vi "3-lorentzian-heat-response -- analytic derivatives.vi"(0 "ζ":dbl(slide)=0.000285 min=0.0 max=0.3 step=1e-06 scale=0.01..10.0 scale format="%#_3p", 1 "T1":dbl(slide)=0.000285 min=0.0 max=0.3 step=1e-06 scale=0.01..10.0 scale format="%#_3p", 2 "τS":dbl(slide)=0.000285 min=0.0 max=0.3 step=1e-06 scale=0.01..10.0 scale format="%#_3p", 3 "τN":dbl(slide)=0.000285 min=0.0 max=0.3 step=1e-06 scale=0.01..10.0 scale format="%#_3p", 4 "τC":dbl(slide)=0.000285 min=0.0 max=0.3 step=1e-06 scale=0.01..10.0 scale format="%#_3p", 5 "κ0":dbl(slide)=0.000285 min=0.0 max=0.3 step=1e-06 scale=0.01..10.0 scale format="%#_3p", 7 "ω (rad/sec)":dbl=0.1 format="%#_10f", 8 "action":T1) -> (13 "R(ω)":cdb=0.1+0.0i format="%#_10f", 14 "d R(ω) / dζ":cdb=-1.0+0.0i, 15 "d R(ω) /  dT1":cdb=-1.0+0.0i, 16 "d R(ω) /  d τS":cdb=-1.0+0.0i, 17 "d R(ω) /  d τN":cdb=-1.0+0.0i, 18 "d R(ω) /  d τC":cdb=-1.0+0.0i, 19 "d R(ω) /  d κ0":cdb=-1.0+0.0i)   [LabVIEW 2020]
uses:
  3-lorentzian-heat-response action.ctl
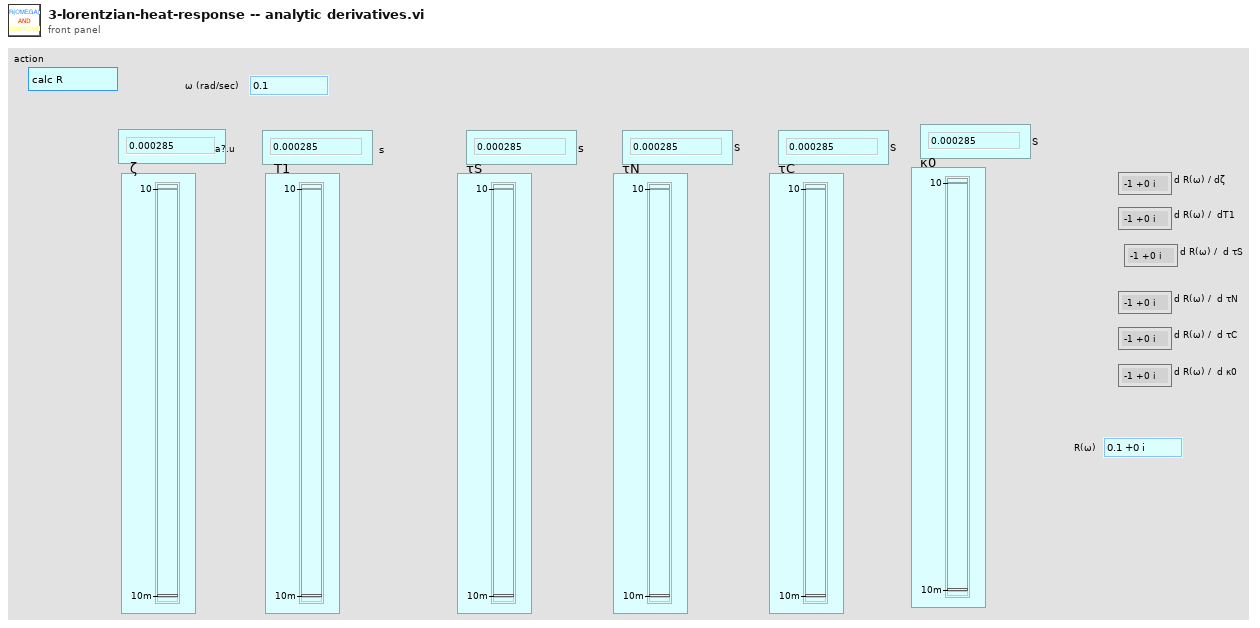
[diagram p1: front panel]
types:
  T1 = typedef "3-lorentzian-heat-response action.ctl" = enum16{"calc R", "create string", "calc m1m2m3", "dζ", "dT1", "dτS", "dτN", "dτC", "d-all", "dκ0"}
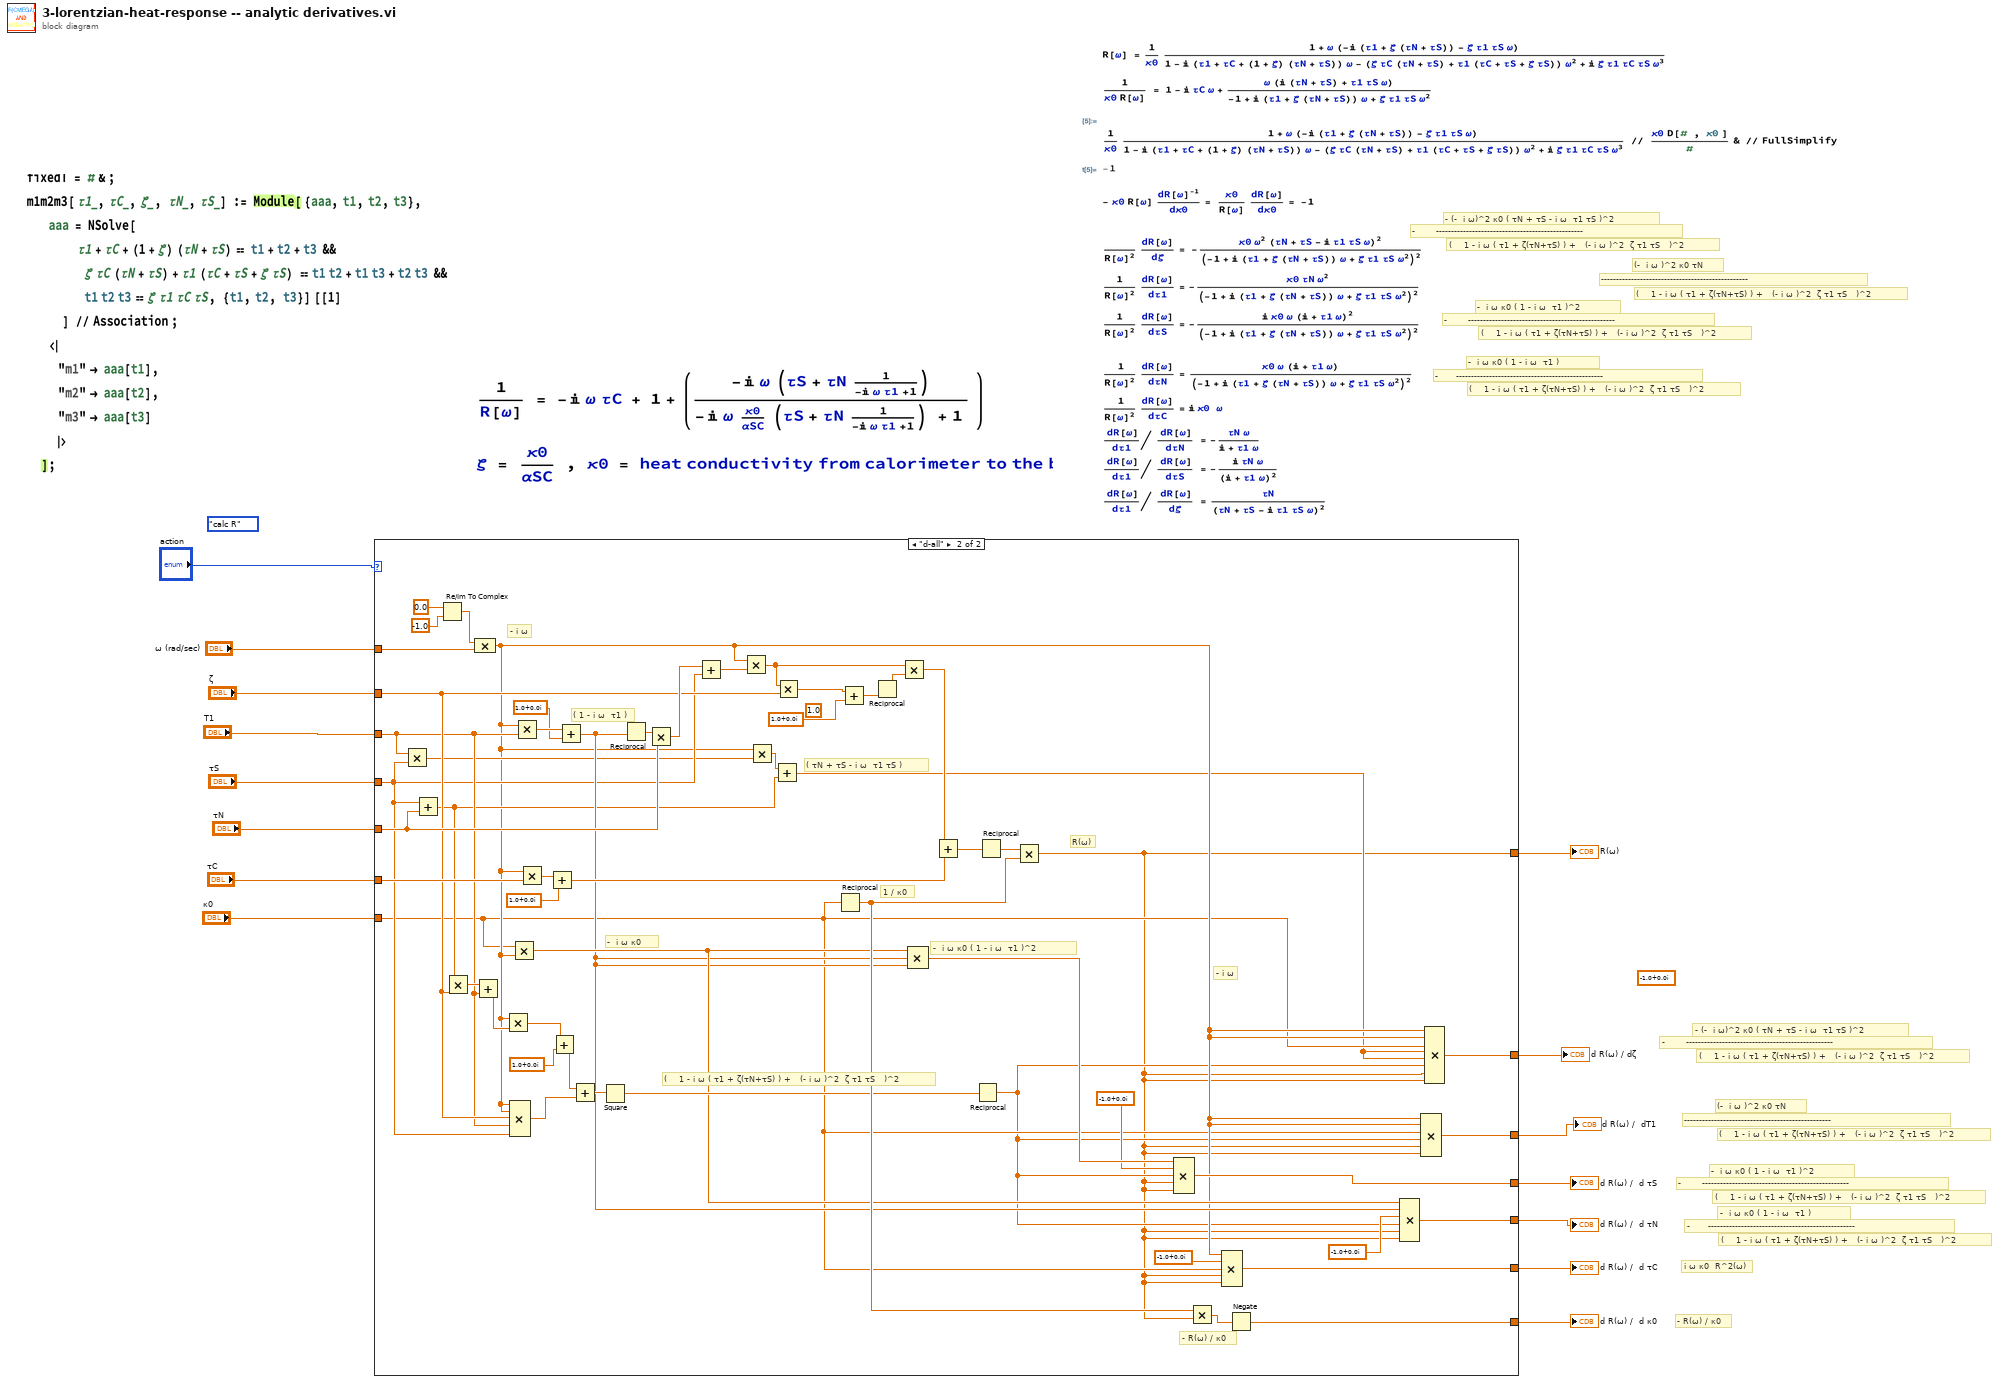
[diagram p0: block diagram]
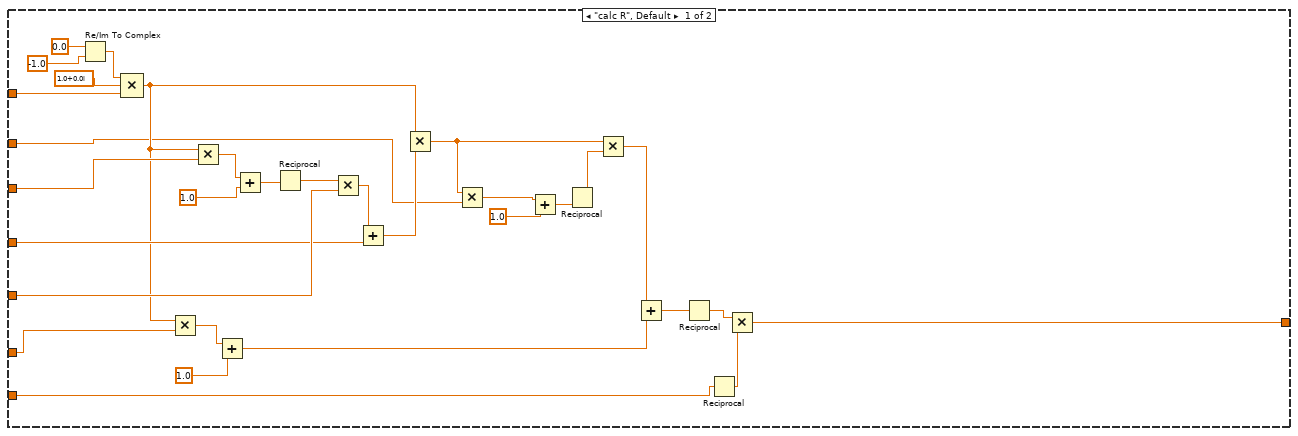
[diagram p2: hidden frame]
diagram:
  (unwired) cdb -1.0+0.0i ("value")
  (unwired) 3-lorentzian-heat-response_action."calc R" ("action")
  # "-       -------------------------------------------------"
  # "- (-  i ω)^2 κ0 ( τN + τS - i ω  τ1 τS )^2"
  # "(    1 - i ω ( τ1 + ζ(τN+τS) ) +   (- i ω )^2  ζ τ1 τS   )^2"
  # "-       -------------------------------------------------"
  # "-  i ω κ0 ( 1 - i ω  τ1 )^2"
  # "(    1 - i ω ( τ1 + ζ(τN+τS) ) +   (- i ω )^2  ζ τ1 τS   )^2"
  # "-------------------------------------------------"
  # "(-  i ω )^2 κ0 τN"
  # "(    1 - i ω ( τ1 + ζ(τN+τS) ) +   (- i ω )^2  ζ τ1 τS   )^2"
  # "-      -------------------------------------------------"
  # "-  i ω κ0 ( 1 - i ω  τ1 )"
  # "(    1 - i ω ( τ1 + ζ(τN+τS) ) +   (- i ω )^2  ζ τ1 τS   )^2"
  # "-       -------------------------------------------------"
  # "- (-  i ω)^2 κ0 ( τN + τS - i ω  τ1 τS )^2"
  # "(    1 - i ω ( τ1 + ζ(τN+τS) ) +   (- i ω )^2  ζ τ1 τS   )^2"
  # "-------------------------------------------------"
  # "(-  i ω )^2 κ0 τN"
  # "(    1 - i ω ( τ1 + ζ(τN+τS) ) +   (- i ω )^2  ζ τ1 τS   )^2"
  # "-      -------------------------------------------------"
  # "-  i ω κ0 ( 1 - i ω  τ1 )"
  # "(    1 - i ω ( τ1 + ζ(τN+τS) ) +   (- i ω )^2  ζ τ1 τS   )^2"
  # "-       -------------------------------------------------"
  # "-  i ω κ0 ( 1 - i ω  τ1 )^2"
  # "(    1 - i ω ( τ1 + ζ(τN+τS) ) +   (- i ω )^2  ζ τ1 τS   )^2"
  # "i ω κ0  R^2(ω)"
  # "- R(ω) / κ0"
  n1 = case shown="\"d-all\"" "action" {
    tunnel: "τC" -> [w32 w94]
    tunnel: "ω (rad/sec)" -> [w35 w96]
    tunnel: "T1" -> [w34 w57]
    tunnel: "τN" -> [w40 w75]
    tunnel: "τS" -> [w38 w56]
    tunnel: "ζ" -> [w28 w70]
    tunnel: [w16 w48] -> w7
    tunnel: "κ0" -> [w19 w51]
    tunnel: [_ w81] -> w6
    tunnel: [_ w79] -> w5
    tunnel: [_ w63] -> w4
    tunnel: [_ w59] -> w3
    tunnel: [_ w58] -> w2
    tunnel: [_ w47] -> w1
    frame "calc R", Default {
      n2 = Re/Im To Complex(1:-1.0 ("y"), 2:0.0 ("x")) -> (0:w36:cdb)
      n3 = Compound Arithmetic op=MULTIPLY(w36, cdb 1.0+0.0i ("value"), w35) -> (w30:cdb)
      n4 = Multiply(x=w30, y=w32) -> (x*y=w31:cdb)
      n5 = Multiply(x=w30, y=w34) -> (x*y=w33:cdb)
      n6 = Add(x=w31, y=1.0) -> (x+y=w22:cdb)
      n7 = Add(x=w33, y=1.0) -> (x+y=w42:cdb)
      n8 = Reciprocal(x=w42) -> (1/x=w41:cdb)
      n9 = Multiply(x=w41, y=w40) -> (x*y=w39:cdb)
      n10 = Add(x=w39, y=w38) -> (x+y=w29:cdb)
      n11 = Multiply(x=w30, y=w29) -> (x*y=w24:cdb)
      n12 = Multiply(x=w24, y=w28) -> (x*y=w26:cdb)
      n13 = Add(x=w26, y=1.0) -> (x+y=w25:cdb)
      n14 = Reciprocal(x=w25) -> (1/x=w23:cdb)
      n15 = Multiply(x=w24, y=w23) -> (x*y=w21:cdb)
      n16 = Add(x=w21, y=w22) -> (x+y=w20:cdb)
      n17 = Reciprocal(x=w20) -> (1/x=w18:cdb)
      n18 = Reciprocal(x=w19) -> (1/x=w17:dbl)
      n19 = Multiply(x=w18, y=w17) -> (x*y=w16:cdb)
    }
    frame "d-all" {
      (unwired) 1.0
      # "( τN + τS - i ω  τ1 τS )"
      # "-  i ω κ0"
      # "( 1 - i ω  τ1 )"
      # "(    1 - i ω ( τ1 + ζ(τN+τS) ) +   (- i ω )^2  ζ τ1 τS   )^2"
      # "-  i ω κ0 ( 1 - i ω  τ1 )^2"
      # "- i ω"
      # "1 / κ0"
      # "- R(ω) / κ0"
      # "- i ω"
      # "R(ω)"
      n20 = Multiply(x=w57, y=w56) -> (x*y=w55:dbl)
      n21 = Add(x=w56, y=w75) -> (x+y=w53:dbl)
      n22 = Re/Im To Complex(1:-1.0 ("y"), 2:0.0 ("x")) -> (0:w97:cdb)
      n23 = Multiply(x=w53, y=w70) -> (x*y=w74:dbl)
      n24 = Add(x=w74, y=w57) -> (x+y=w73:dbl)
      n25 = Compound Arithmetic op=MULTIPLY(w97, w96) -> (w52:cdb)
      n26 = Multiply(x=w52, y=w73) -> (x*y=w72:cdb)
      n27 = Compound Arithmetic op=MULTIPLY(w52, w52, w70, w57, w56) -> (w68:cdb)
      n28 = Multiply(x=w51, y=w52) -> (x*y=w62:cdb)
      n29 = Multiply(x=w52, y=w57) -> (x*y=w95:cdb)
      n30 = Multiply(x=w52, y=w94) -> (x*y=w93:cdb)
      n31 = Add(x=w93, y=cdb 1.0+0.0i ("value")) -> (x+y=w87:cdb)
      n32 = Add(x=w72, y=cdb 1.0+0.0i ("value")) -> (x+y=w69:cdb)
      n33 = Add(x=w95, y=cdb 1.0+0.0i ("value")) -> (x+y=w60:cdb)
      n34 = Add(x=w69, y=w68) -> (x+y=w67:cdb)
      n35 = Square(x=w67) -> (x^2=w64:cdb)
      n36 = Reciprocal(x=w60) -> (1/x=w99:cdb)
      n37 = Multiply(x=w99, y=w75) -> (x*y=w98:cdb)
      n38 = Add(x=w98, y=w56) -> (x+y=w92:cdb)
      n39 = Multiply(x=w52, y=w92) -> (x*y=w89:cdb)
      n40 = Multiply(x=w52, y=w55) -> (x*y=w54:cdb)
      n41 = Add(x=w54, y=w53) -> (x+y=w50:cdb)
      n42 = Multiply(x=w89, y=w70) -> (x*y=w91:cdb)
      n43 = Reciprocal(x=w51) -> (1/x=w83:dbl)
      n44 = Add(x=w91, y=cdb 1.0+0.0i ("value")) -> (x+y=w90:cdb)
      n45 = Reciprocal(x=w90) -> (1/x=w88:cdb)
      n46 = Multiply(x=w89, y=w88) -> (x*y=w86:cdb)
      n47 = Compound Arithmetic op=MULTIPLY(w62, w60, w60) -> (w66:cdb)
      n48 = Add(x=w86, y=w87) -> (x+y=w85:cdb)
      n49 = Reciprocal(x=w64) -> (1/x=w49:cdb)
      n50 = Reciprocal(x=w85) -> (1/x=w84:cdb)
      n51 = Multiply(x=w84, y=w83) -> (x*y=w48:cdb)
      n52 = Compound Arithmetic op=MULTIPLY(w66, cdb -1.0+0.0i ("value"), w49, w48, w48) -> (w63:cdb)
      n53 = Multiply(x=w83, y=w48) -> (x*y=w82:cdb)
      n54 = Compound Arithmetic op=MULTIPLY(w52, cdb -1.0+0.0i ("value"), w51, w48, w48) -> (w79:cdb)
      n55 = Negate(x=w82) -> (-x=w81:cdb)
      n56 = Compound Arithmetic op=MULTIPLY(w62, w60, cdb -1.0+0.0i ("value"), w49, w48, w48) -> (w59:cdb)
      n57 = Compound Arithmetic op=MULTIPLY(w52, w52, w51, w49, w48, w48) -> (w58:cdb)
      n58 = Compound Arithmetic op=MULTIPLY(w52, w52, w51, w50, w50, w49, w48, w48) -> (w47:cdb)
    }
  }
  "R(ω)" <- w7
  "d R(ω) /  d κ0" <- w6
  "d R(ω) /  d τC" <- w5
  "d R(ω) /  d τS" <- w4
  "d R(ω) /  d τN" <- w3
  "d R(ω) /  dT1" <- w2
  "d R(ω) / dζ" <- w1
